vi "AutoDump.vi"(0 "Sample Rate":dbl, 1 "Dump Frequency":dbl, 2 "AutoDump":bool, 3 "AutoLoad":bool, 4 "loopIteration":dbl) -> ()   [LabVIEW 2012]
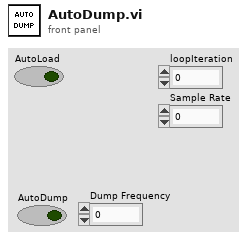
[diagram p1: front panel]
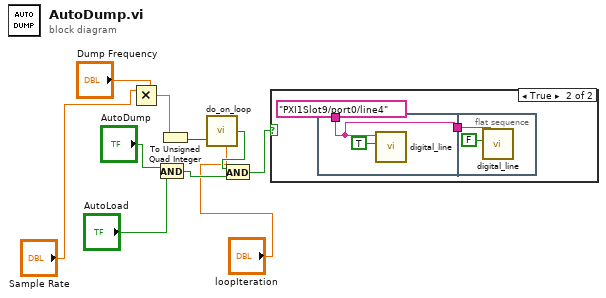
[diagram p0: block diagram]
diagram:
  n1 = Multiply(x="Sample Rate", y="Dump Frequency") -> (x*y=w8:dbl)
  n2 = And(x="AutoDump", y="AutoLoad") -> (x .and. y?=w7:bool)
  n3 = To Unsigned Quad Integer(1:w8) -> (0:w6:u64)
  n4 = call "do_on_loop.vi"("loopsToSkip"=w6, "loopIteration"="loopIteration") -> ("x = 0?"=w5:bool)
  n5 = And(x=w5, y=w7) -> (x .and. y?=w2:bool)
  n6 = case shown="True" w2 {
    frame False {
    }
    frame True {
      n7 = flat-sequence {
        tunnel: tag "PXI1Slot9/port0/line4" ("lines") -> [w14]
        tunnel: [w14] -> w11
        tunnel: w11 -> [w16]
        frame #0 {
          n8 = call "digital_line.vi"("Boolean"=TRUE, "lines"=w14) -> ()  [unwired: 5 in, 1 out]
        }
        frame #1 {
          n9 = call "digital_line.vi"("Boolean"=FALSE, "lines"=w16) -> ()  [unwired: 5 in, 1 out]
        }
      }
    }
  }
